vi "ConversaoPressaokPa.vi"(1 "input":dbl[](array[numeric])) -> (0 "output":dbl[](array[numeric]))   [LabVIEW 2019]
panel:
  out "max":dbl[](array[numeric])
  out "min":dbl[](array[numeric])
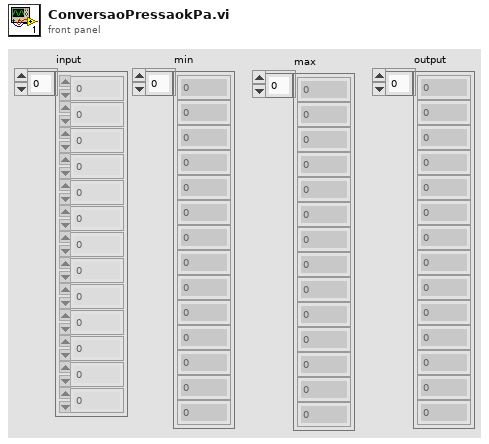
[diagram p1: front panel]
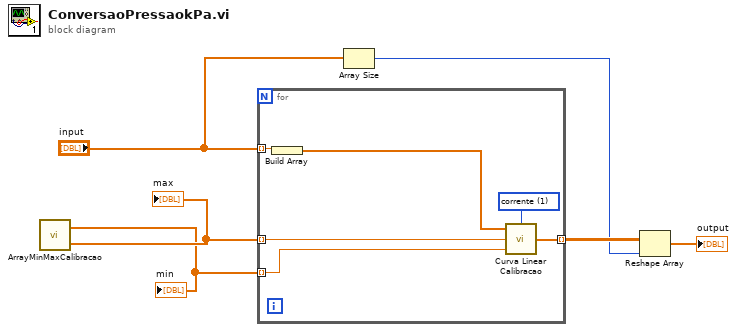
[diagram p0: block diagram]
diagram:
  n1 = call "ArrayMinMaxCalibracao.vi"() -> ("max"=w6:dbl[], "min"=w5:dbl[])  [unwired: 2 in]
  "min" <- w5
  "max" <- w6
  n2 = for {
    tunnel: "input" -> [w11] mode=indexing
    tunnel: w6 -> [w9] mode=indexing
    tunnel: w5 -> [w8] mode=indexing
    tunnel: [w7] -> w4 mode=indexing
    w12 = u16 1 items=["tensao", "corrente"] ("input type")
    n3 = Build Array(w11) -> (w10:dbl[])
    n4 = call "Curva Linear Calibracao.vi"("input type"=w12, "MIN"=w8, "MAX"=w9, "input"=w10) -> ("output"=w7:dbl[])
  }
  n5 = Array Size(array="input") -> (size(s)=w2:i32)
  n6 = Reshape Array(w4, w2) -> (→"output":dbl[])
